vi "Configure Waveform Modifier.vi"(5 "Waveform Modifier (0: Noise)":u16(ring) items=["Noise", "External Signal", "Both"], 6 "Noise Level (10 %)":dbl=10.0 min=0.0 max=50.0 format="%#.6g", 7 "Enable Waveform Modifier (T: Enable)":bool=TRUE, 8 "error in (no error)":errorcluster, 10 "Channel (0: Channel 1)":u16(ring) items=["Channel 1", "Channel 2"], 11 "VISA resource name":refnum<visa-resource-name>) -> (0 "error out":errorcluster, 3 "VISA resource name out":refnum<visa-resource-name>)   [LabVIEW 2019, in "Tektronix AFG 3000 Series.lvlib"]
doc: "Configures whether the function generator adds internal noise, external signal or both to a specified channel."
uses:
  Tektronix AFG 3000 Series.lvlib
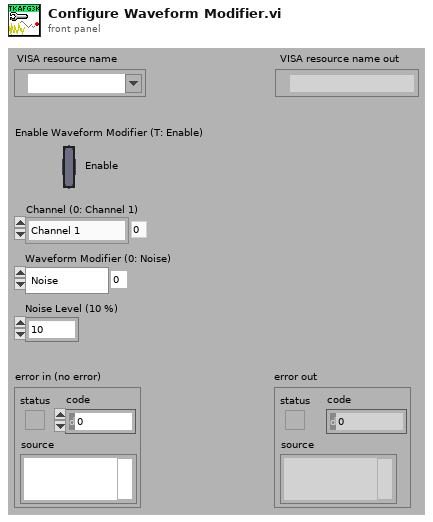
[diagram p1: front panel]
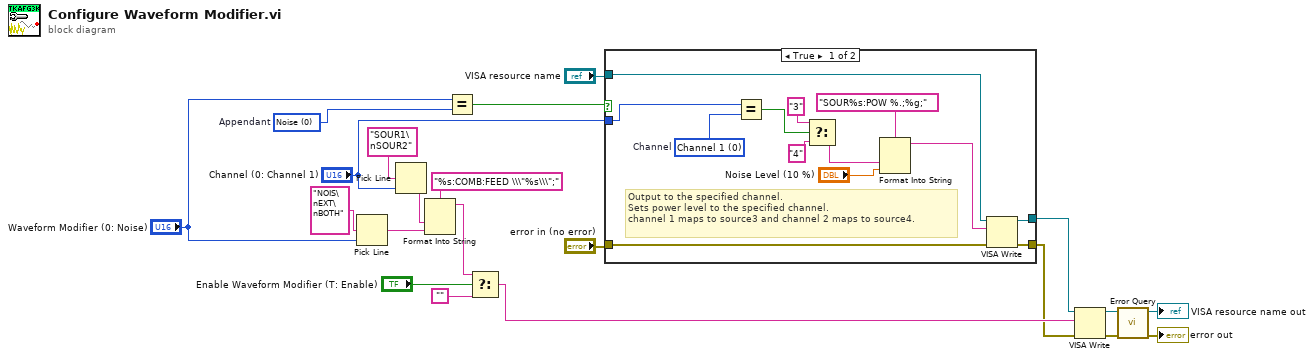
[diagram p0: block diagram]
diagram:
  w10 = u16 0 items=["Noise", "Signal", "Both"]  # Appendant
  n1 = Pick Line(multi-line string="NOIS\nEXT\nBOTH", line index="Waveform Modifier (0: Noise)") -> (output string=w14:string)  [unwired: 1 in]
  n2 = Pick Line(multi-line string="SOUR1\nSOUR2" ("string (\"\")"), line index="Channel (0: Channel 1)") -> (output string=w13:string)  [unwired: 1 in]
  n3 = Format Into String(format string="%s:COMB:FEED \\\"%s\\\";", w13, w14) -> (resulting string=w12:string)  [unwired: 2 in, 1 out]
  n4 = Equal?(x="Waveform Modifier (0: Noise)", y=w10) -> (x = y?=w9:bool)
  n5 = Select(t=w12, s="Enable Waveform Modifier (T: Enable)", f="") -> (s? t:f=w7:string)
  n6 = case shown="True" w9 {
    tunnel: "Channel (0: Channel 1)" -> [w34 _]
    tunnel: "VISA resource name" -> [w25 w35]
    tunnel: "error in (no error)" -> [w27 w36]
    tunnel: [w24 w35] -> w4
    tunnel: [w23 w36] -> w3
    frame True {
      w33 = u16 0 items=["Channel 1", "Channel 2"]  # Channel
      # "Output to the specified channel. \nSets power level to the specified channel.   \nchannel 1 maps to source3 and channel 2 maps to source4."
      n7 = Equal?(x=w34, y=w33) -> (x = y?=w28:bool)
      n8 = Select(t="3" ("format string"), s=w28, f="4" ("format string")) -> (s? t:f=w30:string)
      n9 = Format Into String(format string="SOUR%s:POW %.;%g;", w30, "Noise Level (10 %)") -> (resulting string=w26:string)  [unwired: 2 in, 1 out]
      n10 = VISA Write(VISA resource name=w25, write buffer=w26, error in (no error)=w27) -> (VISA resource name out=w24:refnum<visa-resource-name>, error out=w23:errorcluster)  [unwired: 1 out]
    }
    frame False {
    }
  }
  n11 = VISA Write(VISA resource name=w4, write buffer=w7, error in (no error)=w3) -> (VISA resource name out=w2:refnum<visa-resource-name>, error out=w1:errorcluster)  [unwired: 1 out]
  n12 = call "Error Query.vi"("error in (no error)"=w1, "VISA resource name"=w2) -> ("error out"=→"error out":errorcluster, "VISA resource name out"=→"VISA resource name out":refnum<visa-resource-name>)  [unwired: 6 in, 2 out]
